vi "load correction file.vi"(4 "yoffset":dbl, 5 "xoffset":dbl, 6 "phi":dbl, 7 "ky":dbl, 8 "error in (no error)":errorcluster, 9 "kx":dbl, 10 "cortable":i16, 11 "filename":string) -> (0 "error out":errorcluster, 3 "function return":i16)   [LabVIEW 2015, in "SCANalone4x64.lvlib"]
doc: "__declspec(dllimport) short __stdcall load_correction_file(const char* filename, short cortable, double kx, double ky, double phi, double xoffset, double yoffset);"
uses:
  <userlib>/SCANalone4x64/SCANalone4x64.lvlib
  <userlib>/SCANalone4x64/SCANalone4x64.dll
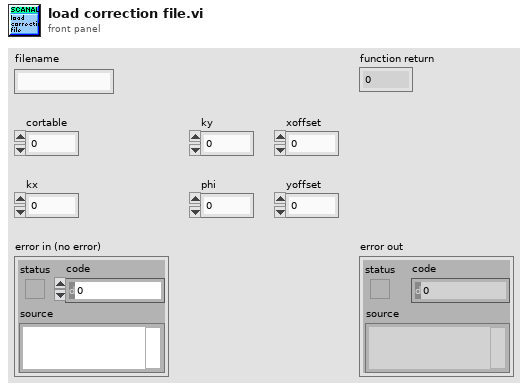
[diagram p1: front panel]
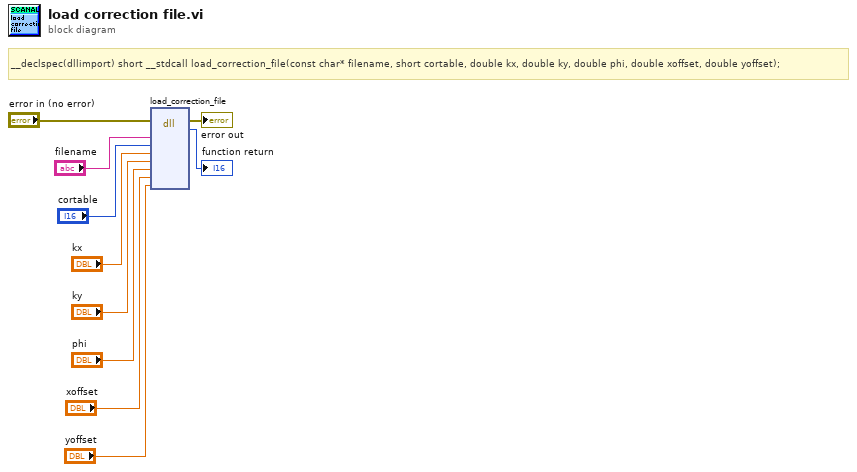
[diagram p0: block diagram]
diagram:
  # "__declspec(dllimport) short __stdcall load_correction_file(const char* filename, short cortable, double kx, double ky, double phi, double xoffset, double yoffset);"
  n1 = dll-call lib="C:/Program Files/National Instruments/LabVIEW 2015/user.lib/SCANalone4x64/SCANalone4x64.*" fn="load_correction_file"(error in="error in (no error)", "filename"="filename", "cortable"="cortable", "kx"="kx", "ky"="ky", "phi"="phi", "xoffset"="xoffset", "yoffset"="yoffset") -> (error out=→"error out":errorcluster, →"function return":i16)  [unwired: 9 in, 1 out]
